vi "hw6p1_hickey.vi"() -> ()   [LabVIEW 2014]
uses:
  <vilib>/imath/engines/lvmath2/RunTimeEngine/Managers/WorkSpace/UID Generator.vi
  <vilib>/imath/engines/lvmath2/RunTimeEngine/RunTimeType/NIMS_RunTimeType_From StrictType (excl LVString).vi
  <instcachedir>/0/NIMS_RunTimeType_From StrictType (excl LVString)_15A5391EEA9C4AACB9955AC755B83D29.lvgen/NIMS_RunTimeType_From StrictType (excl LVString)_15A5391EEA9C4AACB9955AC755B83D29_000.vi
  <vilib>/imath/engines/lvmath2/RunTimeEngine/LocalVariableDefStatement/MC_LocalVariableDefStatement_Display.vi
  <vilib>/imath/engines/lvmath2/RunTimeEngine/VariableToken/NIMS_VariableToken_CondDefined.vi
  <instcachedir>/0/NIMS_VariableToken_CondDefined_EE8DD211A89249938CE6537267F5C9B3.lvgen/NIMS_VariableToken_CondDefined_EE8DD211A89249938CE6537267F5C9B3_005.vi
  <vilib>/imathl/engines/lvmath/Functions/Error Handling/Create Error.vi
  <vilib>/imath/engines/lvmath2/RunTimeEngine/Managers/SymbolTable/Clear UID.vi
  <vilib>/imath/engines/lvmath2/RunTimeEngine/NodeEndStatement/NIMS_NodeEndStatement_Output.vi
  <instcachedir>/0/NIMS_NodeEndStatement_Output_53EC0D466D134D7ABD903AC30B43404B.lvgen/NIMS_NodeEndStatement_Output_53EC0D466D134D7ABD903AC30B43404B_011.vi
  <vilib>/imath/engines/lvmath2/RunTimeEngine/ErrorHandling/NIMS_Finalize Error.vi
  <vilib>/imath/engines/lvmath2/RunTimeEngine/Managers/SymbolTable/NIMS_WorkSpace.lvlib
panel:
  out "Probability of a hit":dbl
  out "Number of hits":dbl
  out "Array":i32[](array[numeric])
  in  "Numeric":i32
  in  "a":dbl
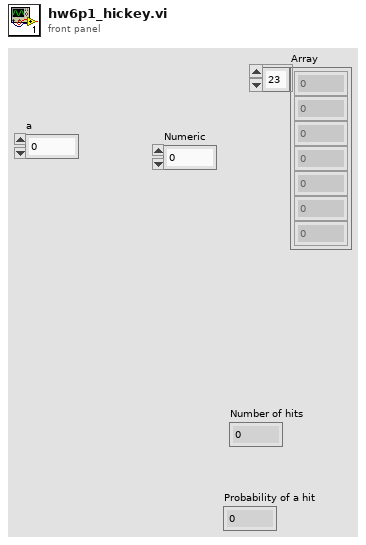
[diagram p1: front panel]
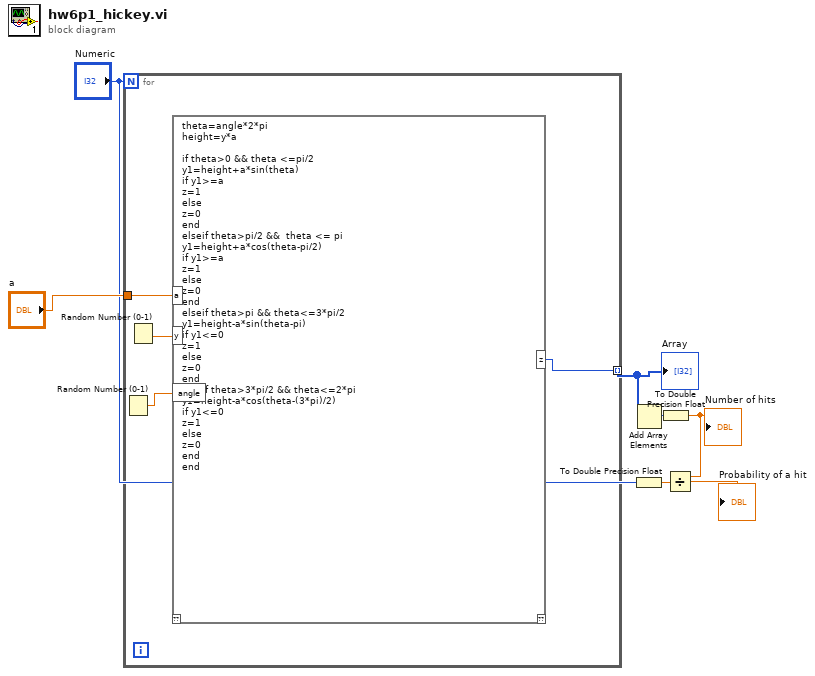
[diagram p0: block diagram]
diagram:
  n1 = for {
    N: "Numeric" -> [_]
    tunnel: "a" -> [w11]
    tunnel: [w8] -> w6 mode=indexing
    n2 = Random Number (0-1)() -> (number: 0 to 1=w10:dbl)
    n3 = Random Number (0-1)() -> (number: 0 to 1=w9:dbl)
    n4 = mathscript code="theta=angle*2*pi\nheight=y*a\n\nif theta>0 && theta <=pi/2\ny1=height+a*sin(theta)\nif y1>=a\nz=1\nelse\nz=0\nend\nelseif theta>pi/2 &&  theta <= pi\ny1=height+a*cos(theta-pi/2)\nif y1>=a\nz=1\nelse\nz=0\nend\nelseif theta>pi && theta<=3*pi/2\ny1=height-a*sin(theta-pi)\nif y1<=0\nz=1\nelse\nz=0\nend\nelseif theta>3*pi/2 && theta<=2*pi\ny1=height-a*cos(theta-(3*pi)/2)\nif y1<=0\nz=1\nelse\nz=0\nend\nend"("a"=w11, "angle"=w10, "y"=w9) -> ("z"=w8:i32)  [unwired: 1 in, 1 out]
  }
  "Array" <- w6
  n5 = Add Array Elements(numeric array=w6) -> (sum=w5:i32)
  n6 = To Double Precision Float(number="Numeric") -> (double precision float=w3:dbl)
  n7 = To Double Precision Float(number=w5) -> (double precision float=w4:dbl)
  "Number of hits" <- w4
  n8 = Divide(x=w4, y=w3) -> (x/y=→"Probability of a hit":dbl)
